vi "Plot Waterfall in Waveform Graph.vi"(4 "total X shift":dbl=1.0 format="%.2f", 6 "total Y shift":dbl=0.5 format="%.2f", 8 "X scale info":cluster{"offset":dbl, "multiplier":dbl}={"offset"=0.0, "multiplier"=1.0} {"multiplier" format="%.2f"; "offset" format="%.2f"}, 9 "Y scale info":cluster{"offset":dbl, "multiplier":dbl}={"offset"=0.0, "multiplier"=1.0} {"multiplier" format="%.2f"; "offset" format="%.2f"}, 10 "Z data":dbl[][](array[numeric]) format="%.2f", 11 "Waterfall Plot":refnum<vi>) -> ()   [LabVIEW 2017]
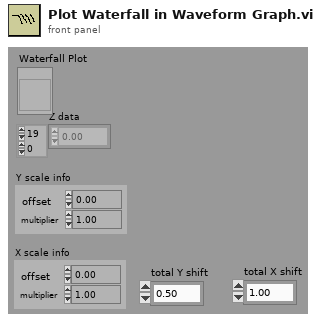
[diagram p1: front panel]
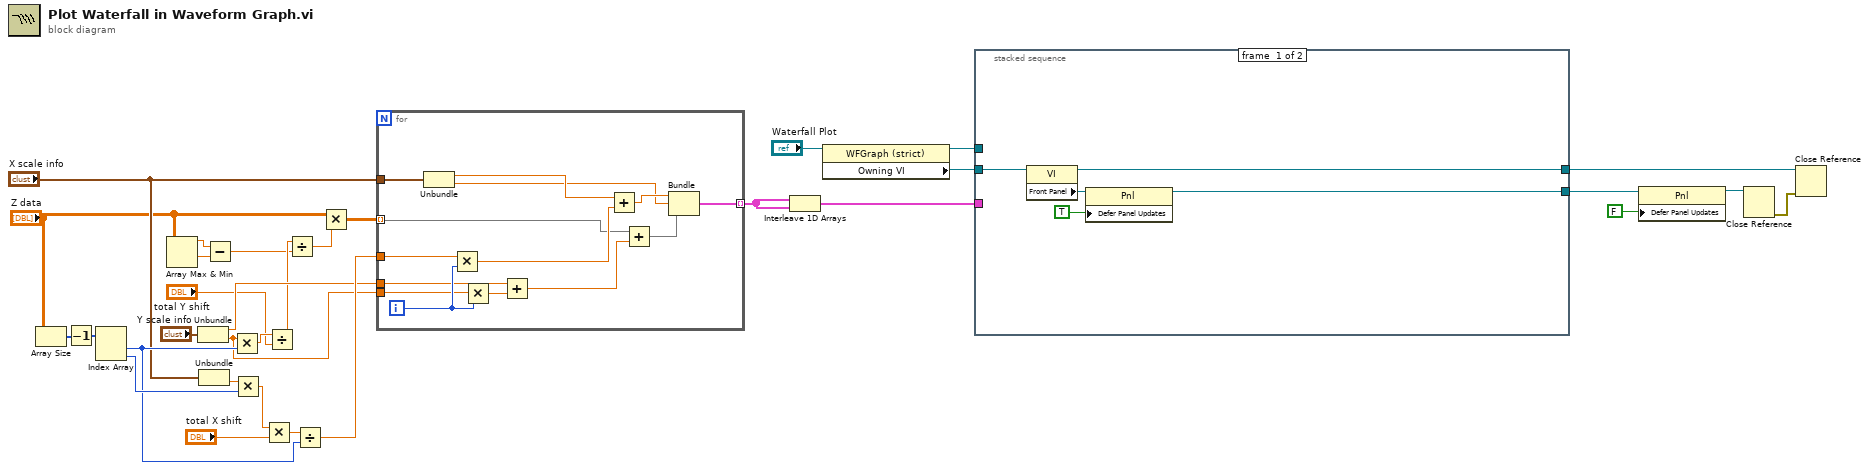
[diagram p0: block diagram]
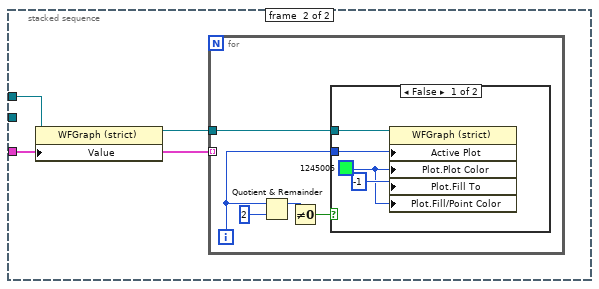
[diagram p2: hidden frame]
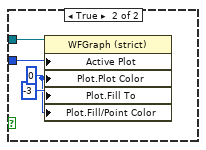
[diagram p3: hidden frame]
diagram:
  n1 = Array Size(array="Z data") -> (size(s)=w32:i32[])
  n2 = Decrement(x=w32) -> (x-1=w30:i32[])
  n3 = Index Array(array=w30) -> (element #1=w24:i32, element #2=w28:i32)  [unwired: 2 in]
  n4 = Array Max & Min(array="Z data") -> (max value=w12:dbl, min value=w14:dbl)  [unwired: 2 out]
  n5 = Unbundle("Y scale info") -> ("offset"=w19:dbl, "multiplier"=w20:dbl)
  n6 = Unbundle("X scale info") -> ("multiplier"=w29:dbl)  [unwired: 1 out]
  n7 = Subtract(x=w12, y=w14) -> (x-y=w13:dbl)
  n8 = Multiply(x=w20, y=w24) -> (x*y=w17:dbl)
  n9 = Multiply(x=w29, y=w28) -> (x*y=w26:dbl)
  n10 = Multiply(x=w26, y="total X shift") -> (x*y=w25:dbl)
  n11 = Divide(x=w17, y="total Y shift") -> (x/y=w15:dbl)
  n12 = Divide(x=w15, y=w13) -> (x/y=w10:dbl)
  n13 = Divide(x=w25, y=w24) -> (x/y=w23:dbl)
  n14 = Multiply(x="Z data", y=w10) -> (x*y=w11:dbl[][])
  n15 = for {
    tunnel: [w42] -> w22 mode=indexing
    tunnel: w11 -> [w38] mode=indexing
    tunnel: "X scale info" -> [w37]
    tunnel: w23 -> [w36]
    tunnel: w20 -> [w35]
    tunnel: w19 -> [w33]
    i -> [w39]
    n16 = Unbundle(w37) -> ("offset"=w41:dbl, "multiplier"=w40:dbl)
    n17 = Multiply(x=w36, y=w39) -> (x*y=w46:dbl)
    n18 = Multiply(x=w35, y=w39) -> (x*y=w45:dbl)
    n19 = Add(x=w33, y=w45) -> (x+y=w34:dbl)
    n20 = Add(x=w41, y=w46) -> (x+y=w43:dbl)
    n21 = Add(x=w38, y=w34) -> (x+y=w44:dbl[])
    n22 = Bundle(w43, "multiplier"=w40, w44) -> (w42:cluster{dbl, "multiplier":dbl, dbl[]})  [unwired: 1 in]
  }
  n23 = Interleave 1D Arrays(w22, w22) -> (w7:cluster{dbl, "multiplier":dbl, dbl[]}[])
  n24 = property class="WFGraph (strict)"(reference="Waterfall Plot") -> (reference out=w8:refnum<vi>, "Owning VI"=w6:refnum<vi>)  [unwired: 1 in, 1 out]
  n25 = stacked-sequence {
    tunnel: w8 -> [_ w53]
    tunnel: w7 -> [_ w52]
    tunnel: w6 -> [w49 _]
    tunnel: [w48 _] -> w4
    tunnel: [w47 _] -> w2
    frame #0 {
      n26 = property class="VI"(reference=w49) -> (reference out=w47:refnum<vi>, "Front Panel"=w50:refnum<vi>)  [unwired: 1 in, 1 out]
      n27 = property class="Pnl"(reference=w50, "Defer Panel Updates"=TRUE) -> (reference out=w48:refnum<vi>)  [unwired: 1 in, 1 out]
    }
    frame #1 {
      n28 = property class="WFGraph (strict)"(reference=w53, "Value"=w52) -> (reference out=w54:refnum<vi>)  [unwired: 1 in, 1 out]
      n29 = for {
        tunnel: w54 -> [w55]
        tunnel: w52 -> [_] mode=indexing
        i -> [w57]
        n30 = Quotient & Remainder(x=w57, y=2) -> (x-y*floor(x/y)=w56:i32)  [unwired: 1 out]
        n31 = Not Equal To 0?(x=w56) -> (x != 0?=w58:bool)
        n32 = case shown="False" w58 {
          tunnel: w57 -> [w62 w67]
          tunnel: w55 -> [w60 w64]
          frame False {
            w61 = u32 1245005
            n33 = property on="Property Node" class="WFGraph (strict)"(reference=w60, "Active Plot"=w62, "Plot.Plot Color"=w61, "Plot.Fill To"=i16 -1, "Plot.Fill/Point Color"=w61) -> ()  [unwired: 1 in, 2 out]
          }
          frame True {
            w65 = u32 0 ("Plot.Plot Color")
            n34 = property on="Property Node" class="WFGraph (strict)"(reference=w64, "Active Plot"=w67, "Plot.Plot Color"=w65, "Plot.Fill To"=i16 -3, "Plot.Fill/Point Color"=w65) -> ()  [unwired: 1 in, 2 out]
          }
        }
      }
    }
  }
  n35 = property class="Pnl"(reference=w4, "Defer Panel Updates"=FALSE) -> (reference out=w3:refnum<vi>)  [unwired: 1 in, 1 out]
  n36 = Close Reference(reference=w3) -> (error out=w1:errorcluster)  [unwired: 1 in]
  n37 = Close Reference(reference=w2, error in (no error)=w1) -> ()  [unwired: 1 out]
